vi "Puff_release2_chs.vi"() -> (5 "Plug in titles":string[](array[string]), 7 "Plug in values":string[](array[string]))   [LabVIEW 2012]
uses:
  Controls/Post_Process.ctl
  Globals/Meas_global.vi
  Globals/Constants_global.vi
  Globals/Dynamic_call_global.ph.vi
  <vilib>/Analysis/NI_AALPro.lvlib
panel:
  in  "PDF samples per block\n(after downsampling)":i32
  in  "Output Directory":path
  in  "Per Block Mode":T1(ring)
  in  "Averaging Samples":i32=1 min=1
  out "Valve trigger Index":dbl format="%.2f"
  out "delay":dbl format="%.2f"
  out "Pulse Width":dbl format="%.2f"
  out "falltime":dbl format="%.2f"
  out "top":dbl format="%.2f"
  out "risetime":dbl format="%.2f"
  in  "Save Time pdf?":bool
  out "Pdf":cluster{"Axis":dbl[], dbl[]}(graph)
  in  "PDF start time (s)":dbl format="%.2f"
  out "Current Block No":i32
  in  "Save averaged traces?":bool
  in  "Pause Mode":T2(ring)
  in  "OK":bool
  out "No of Valid Blocks":dbl
  out "Valve Trace":dbl[](graph)
  out "FFID Trace":cluster{dbl, dbl, dbl[]}(graph)
  out "Valve On":i32
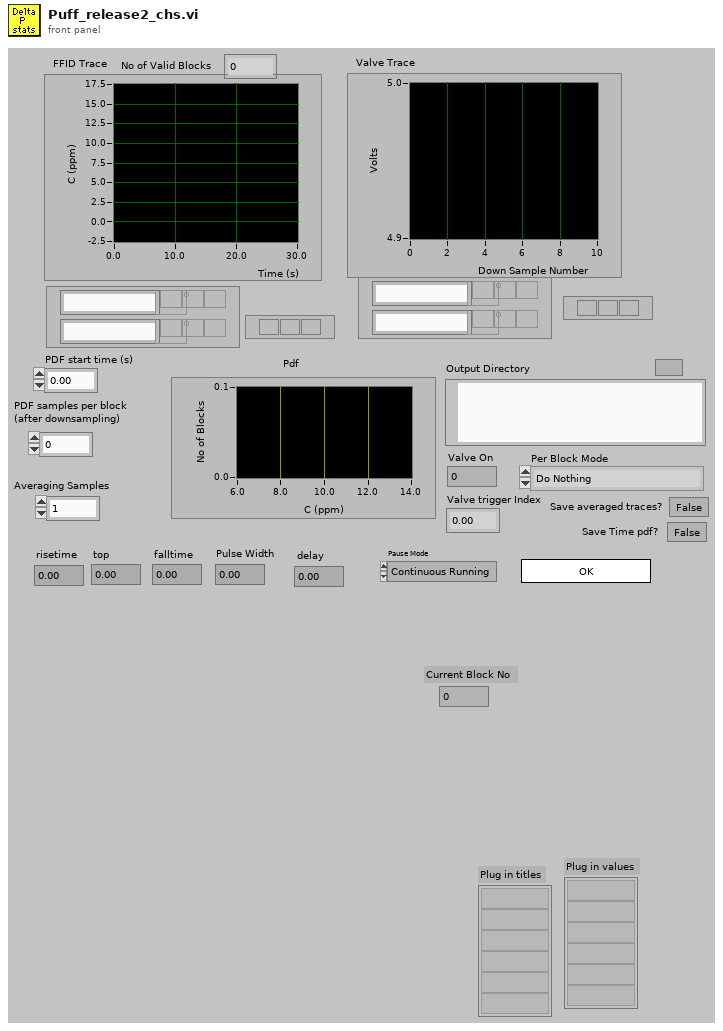
[diagram p1: front panel]
types:
  T1 = enum16{"Do Nothing", "Save Block Time Traces", "Save Jpeg plots"}
  T2 = enum16{"Continuous Running", "After Each  Block"}
  T3 = typedef "Time_Trace_Cluster.ctl" = cluster{"Weighting":dbl[], "Time (s)":dbl[], "Voltage":dbl[], "Eng Values":dbl[]}
  T4 = typedef "Post_Process.ctl" = enum16{"Take New Data", "Post Process Raw Data File"}
  T5 = enum32{"existing file", "new file", "new or existing file", "existing dir", "new dir", "new or existing dir", "existing file (use LLBs)", "new file (use LLBs)", "new or existing file (use LLBs)", "new or existing file or directory (use LLBs)"}
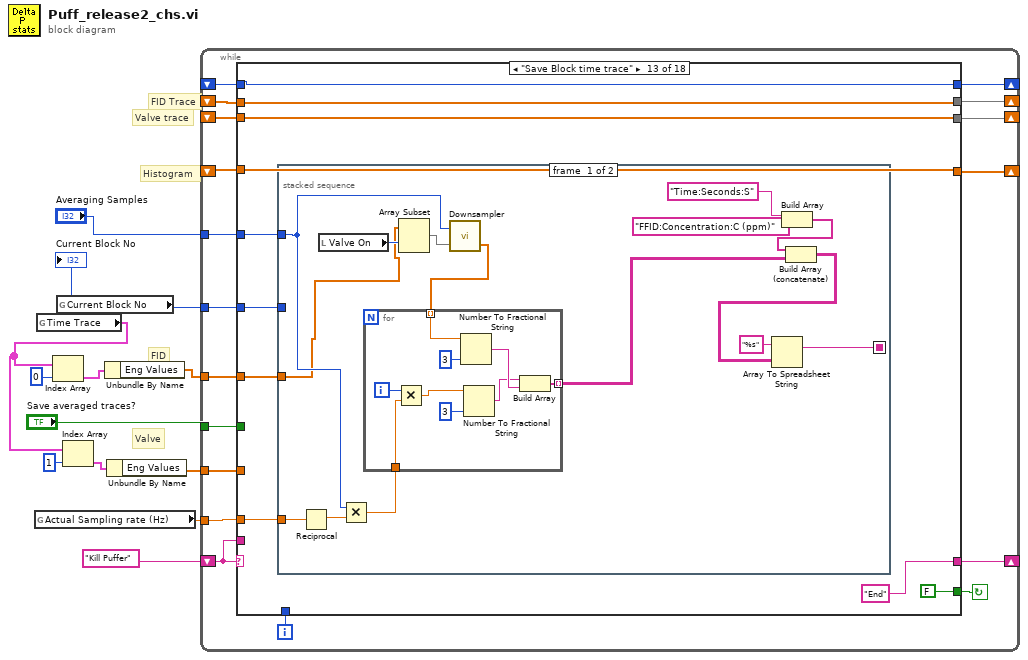
[diagram p0: block diagram]
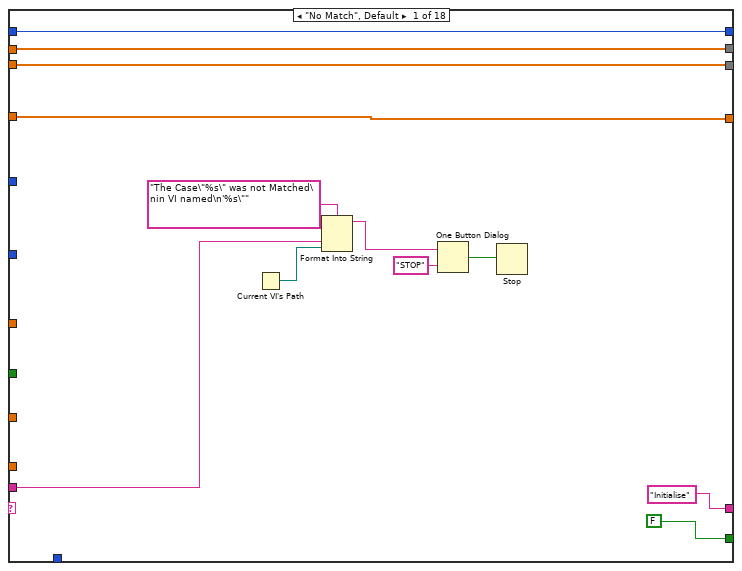
[diagram p2: hidden frame]
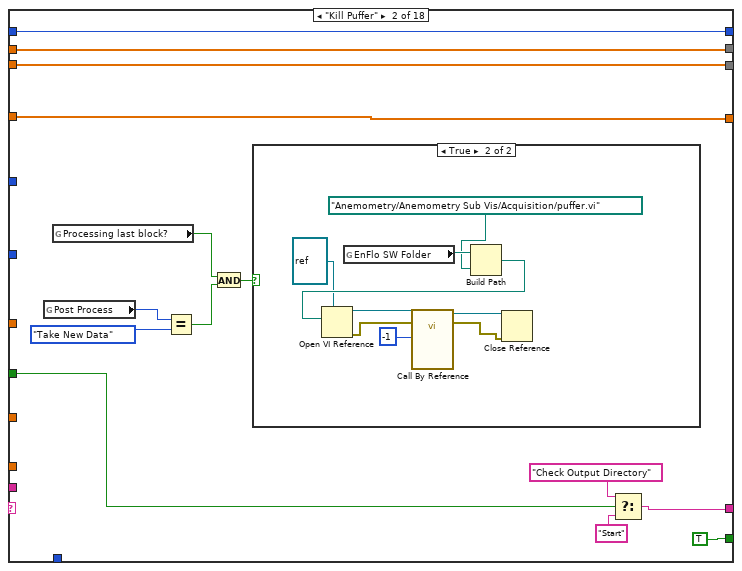
[diagram p3: hidden frame]
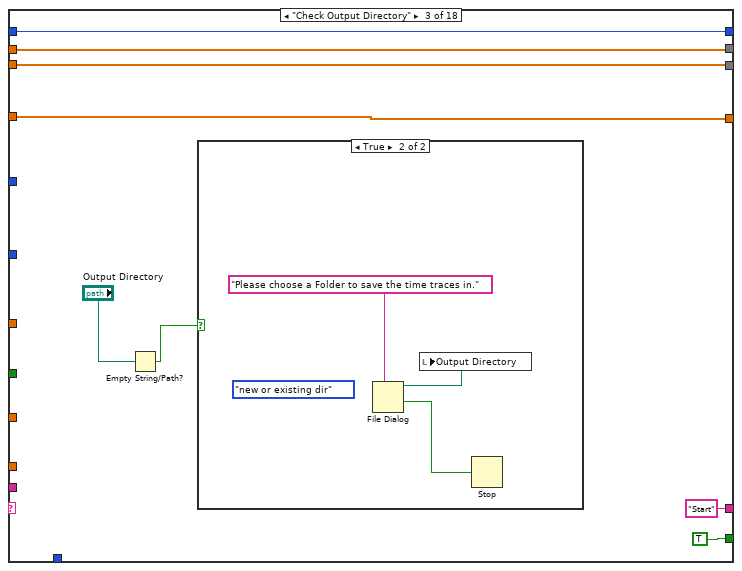
[diagram p5: hidden frame]
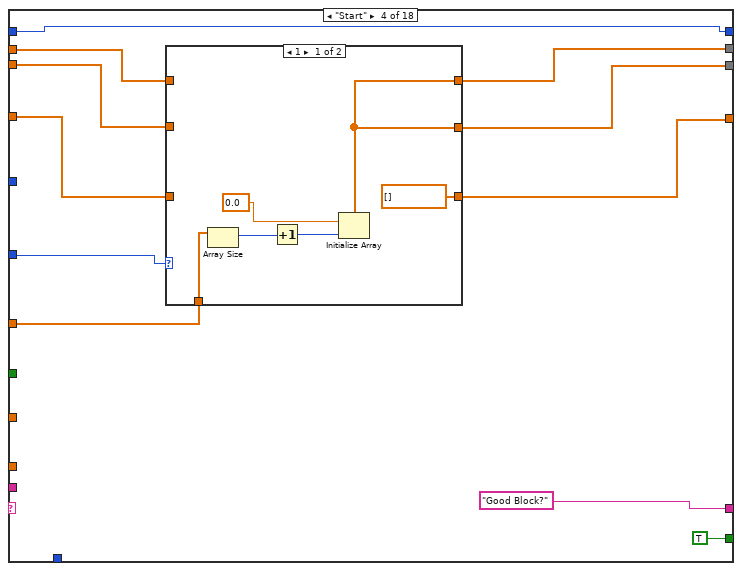
[diagram p7: hidden frame]
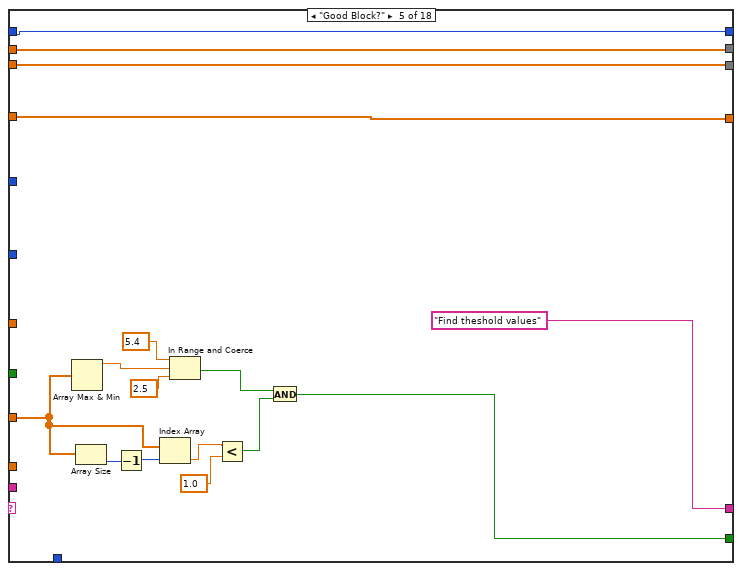
[diagram p9: hidden frame]
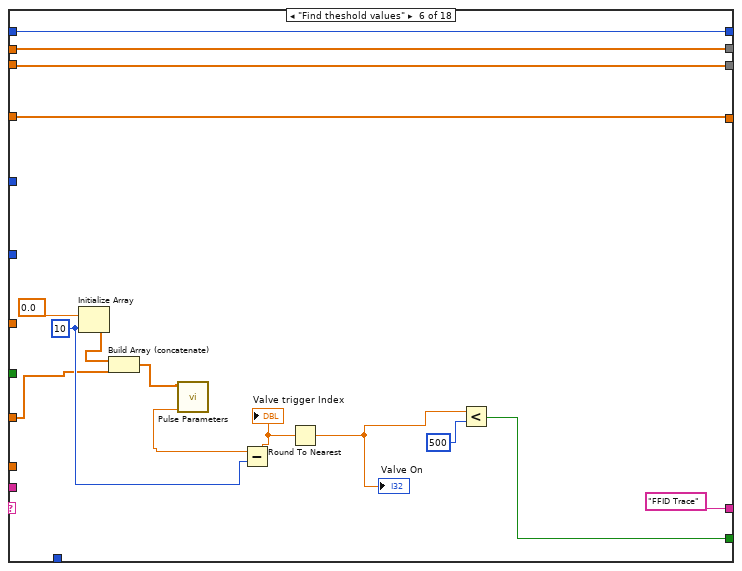
[diagram p10: hidden frame]
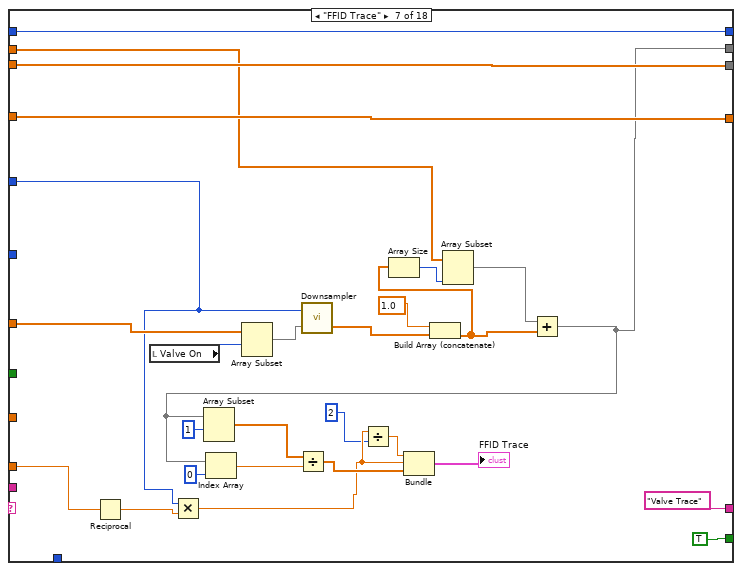
[diagram p11: hidden frame]
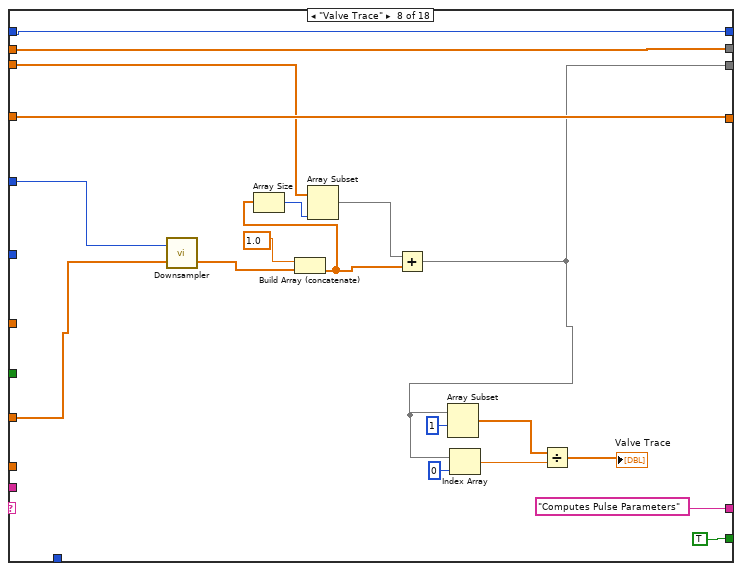
[diagram p12: hidden frame]
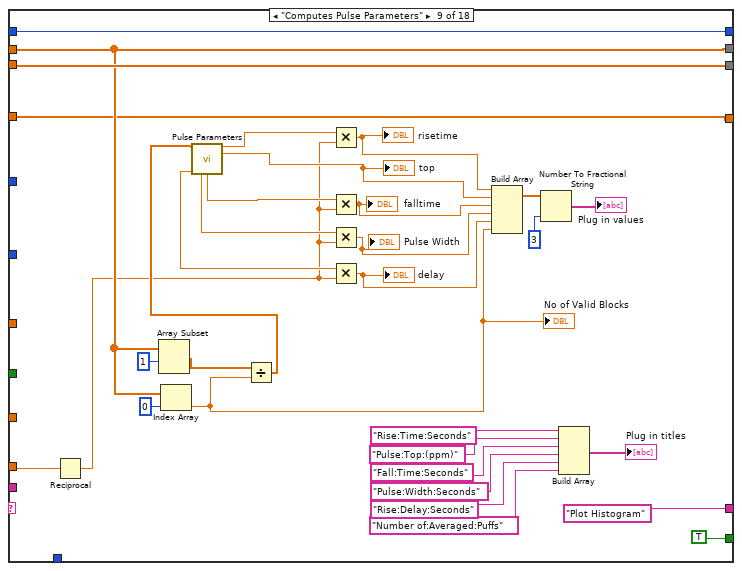
[diagram p13: hidden frame]
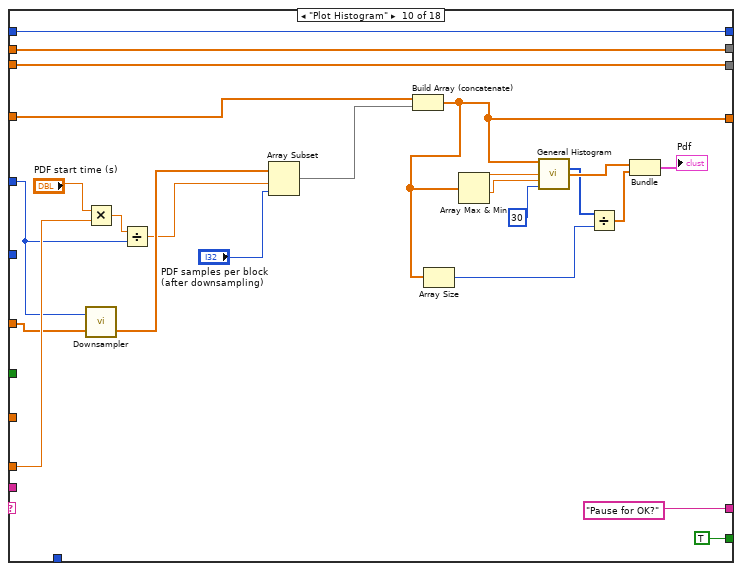
[diagram p14: hidden frame]
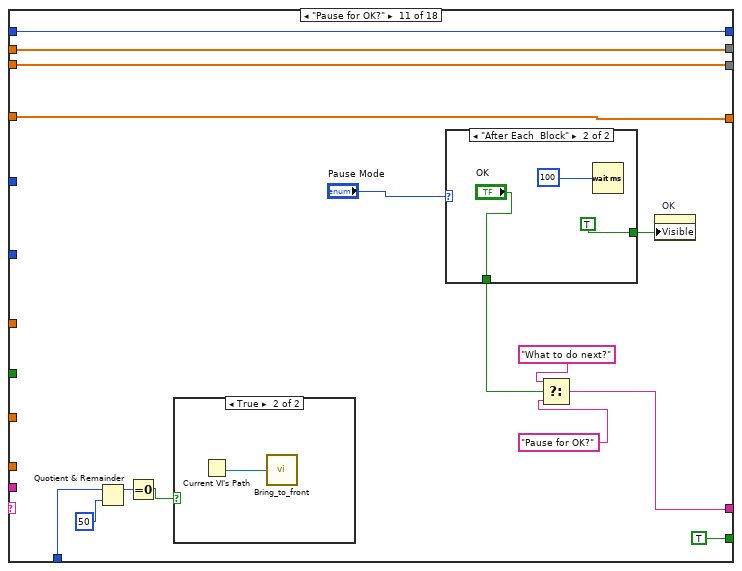
[diagram p15: hidden frame]
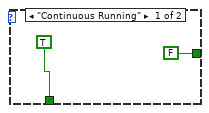
[diagram p17: hidden frame]
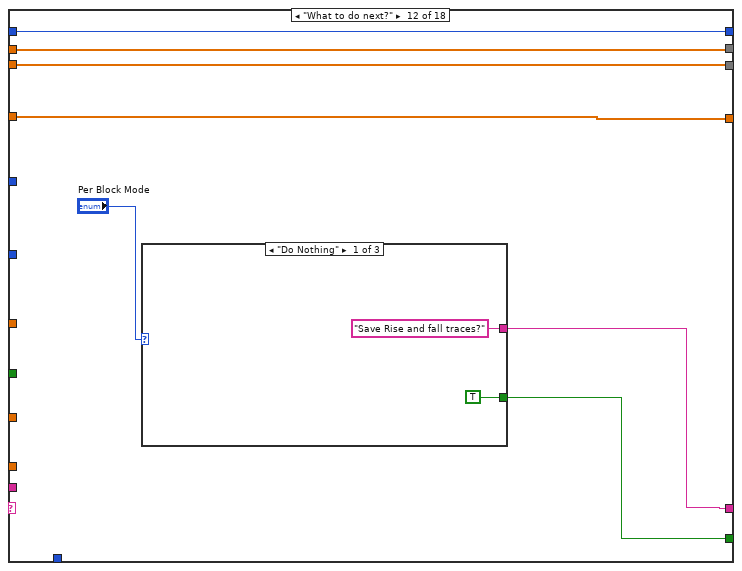
[diagram p18: hidden frame]
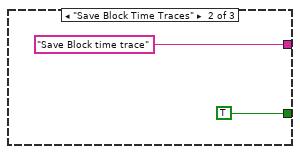
[diagram p19: hidden frame]
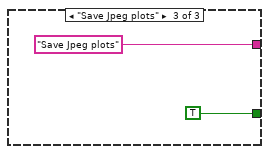
[diagram p20: hidden frame]
diagram:
  # "Valve"
  # "FID"
  # "Histogram"
  # "Valve trace"
  # "FID Trace"
  n1 = global read "Meas_global.vi" "Actual Sampling rate (Hz)"() -> (w11:dbl)
  n2 = global read "Meas_global.vi" "Time Trace"() -> (w5:T3[])
  n3 = Index Array(array=w5, index=0 ("index (row)")) -> (element=w4:T3)
  n4 = global read "Meas_global.vi" "Current Block No"() -> (w10:i32)
  "Current Block No" <- w10
  n5 = Index Array(array=w5, index=1 ("index (row)")) -> (element=w2:T3)
  n6 = Unbundle By Name(w4) -> ("Eng Values"=w3:dbl[])
  n7 = Unbundle By Name(w2) -> ("Eng Values"=w1:dbl[])
  n8 = while {
    shift-left: "Kill Puffer" -> [w28]
    shift-right: [w29] -> _
    shift-right: [w27] -> _
    shift-left: _ -> [w24]
    shift-right: [w26] -> _
    shift-left: _ -> [w25]
    tunnel: w3 -> [w23]
    tunnel: w11 -> [w22]
    tunnel: w10 -> [w21]
    shift-right: [w18] -> _
    shift-left: _ -> [w19]
    shift-right: [w16] -> _
    shift-left: _ -> [w17]
    tunnel: w1 -> [w15]
    tunnel: "Averaging Samples" -> [w14]
    tunnel: "Save averaged traces?" -> [w13]
    i -> [w20]
    stop <- w30 continue-if-true
    n9 = case shown="\"Save Block time trace\"" w28 {
      tunnel: [FALSE TRUE ("Processing last block?") TRUE ("Processing last block?") TRUE ("Processing last block?") w101 w123 TRUE ("Processing last block?") TRUE ("Processing last block?") TRUE ("Processing last block?") TRUE ("Processing last block?") TRUE ("Processing last block?") w251 FALSE ("Processing last block?") FALSE ("Processing last block?") w320 TRUE ("Processing last block?") "Save Time pdf?" FALSE ("Processing last block?")] -> w30
      tunnel: ["Initialise" w43 "Start" "Good Block?" "Find theshold values" "FFID Trace" "Valve Trace" "Computes Pulse Parameters" "Plot Histogram" ("f") "Pause for OK?" ("f") w232 w252 "End" "End" w322 "Save Time pdf?" "Save Time pdf" "End"] -> w29
      tunnel: w28 -> [w37 _ _ _ _ _ _ _ _ _ _ _ _ _ _ _ _ _]
      tunnel: [w34 w56 w73 w86 w112 w126 w143 w171 w176 w229 w244 w257 w273 w318 w327 w334 w409 w417] -> w27
      tunnel: [w33 w55 w72 w84 w111 w125 w152 w155 w203 w228 w243 w256 w272 w317 w326 w333 w408 w416] -> w26
      tunnel: w25 -> [w33 w55 w72 w83 w111 w125 w152 w156 w203 w228 w243 w256 w272 w317 w326 w333 w408 w416]
      tunnel: w24 -> [w34 w56 w73 w85 w112 w126 w132 w171 w176 w229 w244 w257 w273 w318 w327 w334 w409 w417]
      tunnel: w23 -> [_ _ _ w82 _ _ w151 _ _ w210 _ _ w269 w312 _ _ _ w413]
      tunnel: w22 -> [_ _ _ _ _ _ w140 _ w201 w225 _ _ w264 w309 _ _ _ _]
      tunnel: w21 -> [_ _ _ w81 _ _ _ _ _ _ _ _ w268 _ _ _ _ w412]
      tunnel: w20 -> [_ _ _ _ _ _ _ _ _ _ w241 _ _ _ _ _ _ _]
      tunnel: w19 -> [w32 w53 w69 w78 w102 w122 w148 w170 w199 w227 w237 w255 w267 w314 _ w330 _ w411]
      tunnel: [w32 w53 w69 w78 w102 w122 w148 w170 w199 w227 w237 w255 w267 w314 0 w330 0 w411] -> w18
      tunnel: w17 -> [w31 w50 w68 w79 w100 w117 w147 w165 w175 w223 w236 w254 w266 w313 w321 w329 w404 w410]
      tunnel: [w31 w50 w68 w80 w100 w117 w147 w165 w175 w215 w236 w254 w266 w313 w321 w329 w404 w410] -> w16
      tunnel: w15 -> [_ _ _ _ w97 w114 _ w158 _ _ _ _ _ _ _ _ _ _]
      tunnel: w14 -> [_ _ _ _ _ _ w137 w157 _ w207 _ _ w265 _ _ w328 _ _]
      tunnel: w13 -> [_ w46 _ _ _ _ _ _ _ _ _ _ _ _ w319 _ _ _]
      frame "No Match", Default {
        n10 = Current VI's Path() -> (path=w36:path)
        n11 = Format Into String(format string="The Case\"%s\" was not Matched\nin VI named\n'%s\"" ("Format String"), w37, w36) -> (resulting string=w40:string)  [unwired: 2 in, 1 out]
        n12 = One Button Dialog(message=w40, button name ("OK")="STOP") -> (true=w38:bool)
        n13 = Stop(stop? (T)=w38) -> ()
      }
      frame "Kill Puffer" {
        n14 = global read "Meas_global.vi" "Post Process"() -> (w52:T4)
        n15 = global read "Meas_global.vi" "Processing last block?"() -> (w48:bool)
        n16 = Equal?(x=w52, y=Post_Process."Take New Data" ("Post Process")) -> (x = y?=w49:bool)
        n17 = And(x=w48, y=w49) -> (x .and. y?=w47:bool)
        n18 = case shown="True" w47 {
          frame False {
          }
          frame True {
            n19 = global read "Constants_global.vi" "EnFlo SW Folder"() -> (w65:path)
            n20 = Build Path(base path=w65, name or relative path=path "Anemometry/Anemometry Sub Vis/Acquisition/puffer.vi") -> (appended path=w63:path)
            n21 = Open VI Reference(type specifier VI Refnum (for type only)=refnum<vi> refnum, vi path=w63) -> (vi reference=w62:refnum<vi>, error out=w58:errorcluster)  [unwired: 1 in, 3 out]
            n22 = call-by-ref "?"(reference=w62, error in=w58, "number of puffs (cont:0, stop:-1)"=-1) -> (reference out=w59:refnum<vi>, error out=w57:errorcluster)  [unwired: 2 in, 2 out]
            n23 = Close Reference(reference=w59, error in (no error)=w57) -> ()  [unwired: 1 out]
          }
        }
        n24 = Select(t="Check Output Directory", s=w46, f="Start") -> (s? t:f=w43:string)
      }
      frame "Check Output Directory" {
        n25 = Empty String/Path?(string/path="Output Directory") -> (empty?=w67:bool)
        n26 = case shown="True" w67 {
          frame False {
          }
          frame True {
            (unwired) T5."new or existing dir" ("select mode (2)")
            n27 = File Dialog(7:"Please choose a Folder to save the time traces in." ("prompt")) -> (1:w75:bool, 3:w76:path)  [unwired: 1 in, 7 out]
            n28 = local write "Output Directory"(w76) -> ()
            n29 = Stop(stop? (T)=w75) -> ()
          }
        }
      }
      frame "Start" {
        n30 = case shown="1" w81 {
          tunnel: [w89 w96] -> w86
          tunnel: w85 -> [_ w96]
          tunnel: [w89 w95] -> w84
          tunnel: w83 -> [_ w95]
          tunnel: w82 -> [w93 _]
          tunnel: [dbl[] [] w94] -> w80
          tunnel: w79 -> [_ w94]
          frame 1 {
            n31 = Array Size(array=w93) -> (size(s)=w92:i32)
            n32 = Increment(x=w92) -> (x+1=w88:i32)
            n33 = Initialize Array(0.0 ("element"), w88) -> (w89:dbl[])
          }
          frame 2, Default {
          }
        }
      }
      frame "Good Block?" {
        n34 = Array Max & Min(array=w97) -> (max value=w99:dbl)  [unwired: 3 out]
        n35 = Array Size(array=w97) -> (size(s)=w108:i32)
        n36 = Decrement(x=w108) -> (x-1=w107:i32)
        n37 = Index Array(array=w97, index=w107) -> (element=w106:dbl)
        n38 = In Range and Coerce(upper limit=5.4, x=w99, lower limit=2.5 ("y")) -> (In Range?=w103:bool)  [unwired: 1 out]
        n39 = Less?(x=w106, y=1.0) -> (x < y?=w104:bool)
        n40 = And(x=w103, y=w104) -> (x .and. y?=w101:bool)
      }
      frame "Find theshold values" {
        w118 = 10 ("dimension size")
        n41 = Initialize Array(0.0, w118) -> (w119:dbl[])
        n42 = Build Array (concatenate)(w119, w114) -> (w120:dbl[])
        n43 = call <vilib>:"Pulse Parameters.vi"("X"=w120) -> ("delay"=w116:dbl)  [unwired: 14 out]
        n44 = Subtract(x=w116, y=w118) -> (x-y=w115:dbl)
        "Valve trigger Index" <- w115
        n45 = Round To Nearest(number=w115) -> (nearest integer value=w113:dbl)
        "Valve On" <- w113
        n46 = Less?(x=w113, y=500) -> (x < y?=w123:bool)
      }
      frame "FFID Trace" {
        n47 = Reciprocal(x=w140) -> (1/x=w136:dbl)
        n48 = local read "Valve On"() -> (w149:i32)
        n49 = Multiply(x=w137, y=w136) -> (x*y=w130:dbl)
        n50 = Array Subset(array=w151, index=w149) -> (w138:dbl[])  [unwired: 1 in]
        n51 = call "Downsampler.vi"("Input Array"=w138, "Averaging samples"=w137) -> ("Downsampled Array"=w135:dbl[])  [unwired: 1 out]
        n52 = Divide(x=w130, y=2) -> (x/y=w128:dbl)
        n53 = Build Array (concatenate)(1.0, w135) -> (w133:dbl[])
        n54 = Array Size(array=w133) -> (size(s)=w134:i32)
        n55 = Array Subset(array=w132, length=w134) -> (w131:dbl[])  [unwired: 1 in]
        n56 = Add(x=w131, y=w133) -> (x+y=w143:dbl[])
        n57 = Array Subset(array=w143, index=1) -> (w142:dbl[])  [unwired: 1 in]
        n58 = Index Array(array=w143, index=0) -> (element=w141:dbl)
        n59 = Divide(x=w142, y=w141) -> (x/y=w146:dbl[])
        n60 = Bundle(w128, w130, w146) -> (→"FFID Trace":cluster{dbl, dbl, dbl[]})  [unwired: 1 out]
      }
      frame "Valve Trace" {
        n61 = call "Downsampler.vi"("Input Array"=w158, "Averaging samples"=w157) -> ("Downsampled Array"=w162:dbl[])  [unwired: 1 out]
        n62 = Build Array (concatenate)(1.0, w162) -> (w160:dbl[])
        n63 = Array Size(array=w160) -> (size(s)=w161:i32)
        n64 = Array Subset(array=w156, length=w161) -> (w159:dbl[])  [unwired: 1 in]
        n65 = Add(x=w159, y=w160) -> (x+y=w155:dbl[])
        n66 = Array Subset(array=w155, index=1) -> (w167:dbl[])  [unwired: 1 in]
        n67 = Index Array(array=w155, index=0) -> (element=w166:dbl)
        n68 = Divide(x=w167, y=w166) -> (x/y=→"Valve Trace":dbl[])
      }
      frame "Computes Pulse Parameters" {
        n69 = Reciprocal(x=w201) -> (1/x=w174:dbl)
        n70 = Array Subset(array=w176, index=1) -> (w179:dbl[])  [unwired: 1 in]
        n71 = Index Array(array=w176, index=0) -> (element=w178:dbl)
        "No of Valid Blocks" <- w178
        n72 = Divide(x=w179, y=w178) -> (x/y=w177:dbl[])
        n73 = call <vilib>:"Pulse Parameters.vi"("X"=w177) -> ("risetime"=w198:dbl, "top"=w184:dbl, "delay"=w195:dbl, "duration"=w196:dbl, "falltime"=w197:dbl)  [unwired: 10 out]
        "top" <- w184
        n74 = Multiply(x=w198, y=w174) -> (x*y=w183:dbl)
        "risetime" <- w183
        n75 = Multiply(x=w197, y=w174) -> (x*y=w182:dbl)
        "falltime" <- w182
        n76 = Multiply(x=w196, y=w174) -> (x*y=w181:dbl)
        "Pulse Width" <- w181
        n77 = Multiply(x=w195, y=w174) -> (x*y=w180:dbl)
        "delay" <- w180
        n78 = Build Array(w183, w184, w182, w181, w180, w178) -> (w194:dbl[])
        n79 = Number To Fractional String(number=w194, precision (6)=i16 3) -> (F-format string=→"Plug in values":string[])  [unwired: 2 out]
        n80 = Build Array("Rise:Time:Seconds", "Pulse:Top:(ppm)", "Fall:Time:Seconds", "Pulse:Width:Seconds", "Rise:Delay:Seconds", "Number of:Averaged:Puffs") -> (→"Plug in titles":string[])
      }
      frame "Plot Histogram" {
        n81 = Multiply(x="PDF start time (s)", y=w225) -> (x*y=w208:dbl)
        n82 = call "Downsampler.vi"("Input Array"=w210, "Averaging samples"=w207) -> ("Downsampled Array"=w209:dbl[])  [unwired: 1 out]
        n83 = Divide(x=w208, y=w207) -> (x/y=w206:dbl)
        n84 = Array Subset(array=w209, index=w206, length="PDF samples per block\n(after downsampling)") -> (w224:dbl[])
        n85 = Build Array (concatenate)(w223, w224) -> (w215:dbl[])
        n86 = Array Size(array=w215) -> (size(s)=w213:i32)
        n87 = Array Max & Min(array=w215) -> (max value=w222:dbl, min value=w221:dbl)  [unwired: 2 out]
        n88 = call <vilib>:"General Histogram.vi"("X"=w215, "max"=w222, "min"=w221, "# bins"=30) -> ("Histogram"=w214:i32[], "Axis"=w219:dbl[])  [unwired: 2 in, 8 out]
        n89 = Divide(x=w214, y=w213) -> (x/y=w211:dbl[])
        n90 = Bundle("Axis"=w219, w211) -> (→"Pdf":cluster{"Axis":dbl[], dbl[]})  [unwired: 1 out]
      }
      frame "Pause for OK?" {
        n91 = Quotient & Remainder(x=w241, y=50) -> (x-y*floor(x/y)=w239:i32)  [unwired: 1 out]
        n92 = Equal To 0?(x=w239) -> (x = 0?=w238:bool)
        n93 = case shown="True" w238 {
          frame False {
          }
          frame True {
            n94 = Current VI's Path() -> (path=w245:path)
            n95 = call "Bring_to_front.vi"("path"=w245) -> ()
          }
        }
        n96 = case shown="\"After Each  Block\"" "Pause Mode" {
          tunnel: [TRUE "OK"] -> w233
          tunnel: [FALSE TRUE] -> w242
          frame "Continuous Running" {
          }
          frame "After Each  Block" {
            n97 = Wait (ms)(milliseconds to wait=u32 100 ("f")) -> ()  [unwired: 1 out]
          }
        }
        n98 = Select(t="What to do next?" ("f"), s=w233, f="Pause for OK?") -> (s? t:f=w232:string)
        n99 = property on="OK" class="Bool"("Visible"=w242) -> ()  [unwired: 2 in, 2 out]
      }
      frame "What to do next?" {
        n100 = case shown="\"Do Nothing\"" "Per Block Mode" {
          tunnel: ["Save Rise and fall traces?" ("t") "Save Block time trace" ("t") "Save Jpeg plots" ("t")] -> w252
          tunnel: [TRUE TRUE TRUE] -> w251
          frame "Do Nothing" {
          }
          frame "Save Block Time Traces" {
          }
          frame "Save Jpeg plots" {
          }
        }
      }
      frame "Save Block time trace" {
        n101 = stacked-sequence {
          seq-local: [w283 _] -> [_ w303]
          tunnel: w269 -> [w274 _]
          tunnel: w268 -> [_ w301]
          tunnel: w265 -> [w276 _]
          tunnel: w264 -> [w278 _]
          frame #0 {
            n102 = Reciprocal(x=w278) -> (1/x=w277:dbl)
            n103 = local read "Valve On"() -> (w281:i32)
            n104 = Multiply(x=w276, y=w277) -> (x*y=w275:dbl)
            n105 = Array Subset(array=w274, index=w281) -> (w280:dbl[])  [unwired: 1 in]
            n106 = call "Downsampler.vi"("Input Array"=w280, "Averaging samples"=w276) -> ("Downsampled Array"=w279:dbl[])  [unwired: 1 out]
            n107 = for {
              tunnel: [w295] -> w282 mode=indexing
              tunnel: w279 -> [w292] mode=indexing
              tunnel: w275 -> [w291]
              i -> [w290]
              n108 = Multiply(x=w290, y=w291) -> (x*y=w289:dbl)
              n109 = Number To Fractional String(number=w292, precision (6)=i16 3) -> (F-format string=w294:string)  [unwired: 2 out]
              n110 = Number To Fractional String(number=w289, precision (6)=i16 3) -> (F-format string=w293:string)  [unwired: 2 out]
              n111 = Build Array(w293, w294) -> (w295:string[])
            }
            n112 = Build Array("Time:Seconds:S", "FFID:Concentration:C (ppm)") -> (w286:string[])
            n113 = Build Array (concatenate)(w286, w282) -> (w285:string[][])
            n114 = Array To Spreadsheet String(array=w285, 3:"%s" ("format string")) -> (spreadsheet string=w283:string)  [unwired: 1 out]
          }
          frame #1 {
            w305 = TRUE  # advisory dialog? (display:T)
            n115 = global read "Meas_global.vi" "Raw data file"() -> (w308:path)
            n116 = Strip Path(path=w308) -> (name=w302:string)  [unwired: 1 out]
            n117 = local read "Output Directory"() -> (w298:path)
            n118 = Format Into String(format string="_B%d", initial string=w302, w301) -> (resulting string=w299:string)  [unwired: 1 in, 1 out]
            n119 = Build Path(base path=w298, name or relative path=w299) -> (appended path=w307:path)
            n120 = call "Find_Unique_Filename.vi"("Path In"=w307) -> ("Unique Path Out"=w306:path)  [unwired: 1 in, 1 out]
            n121 = call "Write_Characters_To_File.vi"("file path (dialog if empty)"=w306, "advisory dialog? (display:T)"=w305, "character string"=w303, "append to file? (new file:F)"=FALSE) -> ()  [unwired: 1 in, 4 out]
          }
        }
      }
      frame "Save Jpeg plots" {
        n122 = local read "Valve On"() -> (w311:i32)
        n123 = Array Subset(array=w312, index=w311) -> (w310:dbl[])  [unwired: 1 in]
        n124 = call "Puff_realisation_display.vi"("Actual Sampling rate (Hz)"=w309, "Input Array"=w310) -> ()  [unwired: 2 out]
      }
      frame "Save Rise and fall traces?" {
        n125 = Select(t="Save averaged time trace", s=w319, f="Save Time PDF?") -> (s? t:f=w322:string)
        n126 = global read "Meas_global.vi" "Processing last block?"() -> (w320:bool)
      }
      frame "Save averaged time trace" {
        n127 = stacked-sequence {
          seq-local: [w347 _] -> [_ w382]
          tunnel: w328 -> [w337 _]
          frame #0 {
            n128 = local read "FFID Trace"() -> (w356:cluster{dbl, dbl, dbl[]})
            n129 = local read "Valve On"() -> (w336:i32)
            n130 = local read "Valve Trace"() -> (w340:dbl[])
            n131 = Unbundle(w356) -> (w354:dbl, w355:dbl, w338:dbl[])
            n132 = Divide(x=w336, y=w337) -> (x/y=w335:dbl)
            n133 = Array Subset(array=w340, index=w335) -> (w339:dbl[])  [unwired: 1 in]
            n134 = for {
              tunnel: w355 -> [w367]
              tunnel: w354 -> [w366]
              tunnel: w338 -> [w361] mode=indexing
              tunnel: [w364] -> w352 mode=indexing
              tunnel: w339 -> [w362] mode=indexing
              i -> [w368]
              n135 = Multiply(x=w367, y=w368) -> (x*y=w365:dbl)
              n136 = Add(x=w366, y=w365) -> (x+y=w363:dbl)
              n137 = Build Array(w363, w362, w361) -> (w364:dbl[])
            }
            n138 = Build Array("Time:(s):T=0 when valve opened", "Source:Valve:Voltage", "FFID:Concentration:C") -> (w344:string[])
            n139 = for {
              tunnel: w344 -> [w360] mode=indexing
              tunnel: [w359] -> w343 mode=indexing
              tunnel: [w358] -> w342 mode=indexing
              tunnel: [w357] -> w341 mode=indexing
              n140 = call "Split_Ch_name.vi"("Ch name"=w360) -> ("Top level"=w359:string, "Middle"=w358:string, "Low level"=w357:string)
            }
            n141 = Number To Fractional String(number=w352, precision (6)=i16 3) -> (F-format string=w351:string[][])  [unwired: 2 out]
            n142 = Build Array (concatenate)(w343, w342, w341, w351) -> (w349:string[][])
            n143 = Array To Spreadsheet String(array=w349, 3:"%s" ("format string")) -> (spreadsheet string=w347:string)  [unwired: 1 out]
          }
          frame #1 {
            w394 = TRUE  # advisory dialog? (display:T)
            n144 = local read "No of Valid Blocks"() -> (w370:dbl)
            n145 = global read "Meas_global.vi" "Raw data file"() -> (w399:path)
            n146 = global read "Dynamic_call_global.ph.vi" "Plug in titles"() -> (w375:string[])
            n147 = global read "Dynamic_call_global.ph.vi" "Plug in values"() -> (w372:string[])
            n148 = Strip Path(path=w399) -> (name=w380:string)  [unwired: 1 out]
            n149 = String Subset(string=w380, offset (0)=0, length (rest)=28 ("length (rest)")) -> (substring=w377:string)
            n150 = Number To Decimal String(number=w370) -> (decimal integer string=w369:string)  [unwired: 1 out]
            n151 = Build Array (concatenate)("No of:Blocks:Processed", w375) -> (w373:string[])
            n152 = Build Array (concatenate)(w369, w372) -> (w371:string[])
            n153 = local read "Output Directory"() -> (w376:path)
            n154 = for {
              tunnel: w373 -> [w403] mode=indexing
              tunnel: [w402] -> w392 mode=indexing
              tunnel: [w401] -> w391 mode=indexing
              tunnel: [w400] -> w390 mode=indexing
              n155 = call "Split_Ch_name.vi"("Ch name"=w403) -> ("Top level"=w402:string, "Middle"=w401:string, "Low level"=w400:string)
            }
            n156 = Concatenate Strings(w377, "_P" ("string")) -> (w398:string)
            n157 = Initialize Array("", 15) -> (w387:string[])
            n158 = Build Path(base path=w376, name or relative path=w398) -> (appended path=w396:path)
            n159 = call "Asterisk_header.vi"("Channel names"=w387) -> ("Header string"=w383:string)
            n160 = call "Find_Unique_Filename.vi"("Path In"=w396) -> ("Unique Path Out"=w395:path)  [unwired: 1 in, 1 out]
            n161 = Build Array(w392, w391, w390, w371) -> (w388:string[][])
            n162 = Array To Spreadsheet String(array=w388, 3:"%s" ("format string")) -> (spreadsheet string=w384:string)  [unwired: 1 out]
            n163 = Concatenate Strings(w384, w383, w382) -> (w381:string)
            n164 = call "Write_Characters_To_File.vi"("file path (dialog if empty)"=w395, "advisory dialog? (display:T)"=w394, "character string"=w381, "append to file? (new file:F)"=FALSE) -> ()  [unwired: 1 in, 4 out]
          }
        }
      }
      frame "Save Time pdf?" {
      }
      frame "Save Time pdf" {
        n165 = stacked-sequence {
          seq-local: [w428 _] -> [_ w461]
          tunnel: w413 -> [_ _]
          tunnel: w412 -> [_ _]
          frame #0 {
            n166 = local read "Pdf"() -> (w426:cluster{"Axis":dbl[], dbl[]})
            n167 = Unbundle(w426) -> ("Axis"=w425:dbl[], w424:dbl[])
            n168 = for {
              tunnel: w424 -> [w439] mode=indexing
              tunnel: w425 -> [w446] mode=indexing
              tunnel: [w445] -> w427 mode=indexing
              shift-right: [w438] -> _
              shift-left: 0.0 -> [w440]
              n169 = Add(x=w439, y=w440) -> (x+y=w438:dbl)
              n170 = Number To Fractional String(number=w439, precision (6)=i16 3) -> (F-format string=w443:string)  [unwired: 2 out]
              n171 = Number To Fractional String(number=w438, precision (6)=i16 3) -> (F-format string=w437:string)  [unwired: 2 out]
              n172 = Number To Fractional String(number=w446, precision (6)=i16 3) -> (F-format string=w444:string)  [unwired: 2 out]
              n173 = Build Array(w444, w443, w437) -> (w445:string[])
            }
            n174 = Build Array("FFID:Concentration:C (ppm)", "Pdf:Bin:Frequency", "Cumulative Pdf:Bin:Frequency") -> (w423:string[])
            n175 = for {
              tunnel: w423 -> [w436] mode=indexing
              tunnel: [w435] -> w422 mode=indexing
              tunnel: [w434] -> w421 mode=indexing
              tunnel: [w433] -> w420 mode=indexing
              n176 = call "Split_Ch_name.vi"("Ch name"=w436) -> ("Top level"=w435:string, "Middle"=w434:string, "Low level"=w433:string)
            }
            n177 = Build Array (concatenate)(w422, w421, w420, w427) -> (w430:string[][])
            n178 = Array To Spreadsheet String(array=w430, 3:"%s" ("format string")) -> (spreadsheet string=w428:string)  [unwired: 1 out]
          }
          frame #1 {
            w476 = TRUE  # advisory dialog? (display:T)
            n179 = global read "Dynamic_call_global.ph.vi" "Plug in titles"() -> (w450:string[])
            n180 = global read "Dynamic_call_global.ph.vi" "Plug in values"() -> (w452:string[])
            n181 = local read "No of Valid Blocks"() -> (w454:dbl)
            n182 = global read "Meas_global.vi" "Raw data file"() -> (w479:path)
            n183 = local read "PDF start time (s)"() -> (w472:dbl)
            n184 = Strip Path(path=w479) -> (name=w457:string)  [unwired: 1 out]
            n185 = Build Array (concatenate)("No of:Blocks:Processed", w450) -> (w449:string[])
            n186 = Number To Decimal String(number=w454) -> (decimal integer string=w453:string)  [unwired: 1 out]
            n187 = Build Array (concatenate)(w453, w452) -> (w451:string[])
            n188 = String Subset(string=w457, offset (0)=0, length (rest)=20 ("length (rest)")) -> (substring=w456:string)
            n189 = for {
              tunnel: w449 -> [w483] mode=indexing
              tunnel: [w482] -> w471 mode=indexing
              tunnel: [w481] -> w470 mode=indexing
              tunnel: [w480] -> w469 mode=indexing
              n190 = call "Split_Ch_name.vi"("Ch name"=w483) -> ("Top level"=w482:string, "Middle"=w481:string, "Low level"=w480:string)
            }
            n191 = Format Into String(format string="_T=%d", initial string=w456, w472) -> (resulting string=w473:string)  [unwired: 1 in, 1 out]
            n192 = local read "Output Directory"() -> (w455:path)
            n193 = Initialize Array("", 15) -> (w466:string[])
            n194 = Build Path(base path=w455, name or relative path=w473) -> (appended path=w478:path)
            n195 = call "Asterisk_header.vi"("Channel names"=w466) -> ("Header string"=w462:string)
            n196 = call "Find_Unique_Filename.vi"("Path In"=w478) -> ("Unique Path Out"=w477:path)  [unwired: 1 in, 1 out]
            n197 = Build Array(w471, w470, w469, w451) -> (w467:string[][])
            n198 = Array To Spreadsheet String(array=w467, 3:"%s" ("format string")) -> (spreadsheet string=w463:string)  [unwired: 1 out]
            n199 = Concatenate Strings(w463, w462, w461) -> (w460:string)
            n200 = call "Write_Characters_To_File.vi"("file path (dialog if empty)"=w477, "advisory dialog? (display:T)"=w476, "character string"=w460, "append to file? (new file:F)"=FALSE) -> ()  [unwired: 1 in, 4 out]
          }
        }
      }
    }
  }
